vi "DSF.Shared.Configuration.Transfer.Get Engine Offset.vi"(11 "Transfer Configuration in":refnum<class "DSF.Shared.Configuration.Transfer.lvclass">) -> (2 "engine offset":u64, 3 "Transfer Configuration out":refnum<class "DSF.Shared.Configuration.Transfer.lvclass">)   [LabVIEW 2017, in "DSF.Engine.lvlib" / "DSF.Shared.Configuration.Transfer.lvclass"]
uses:
  DSF.Shared.Configuration.Transfer.lvclass
  DSF.Shared.Configuration.Transfer.lvclass/DSF.Shared.Configuration.Transfer.ctl
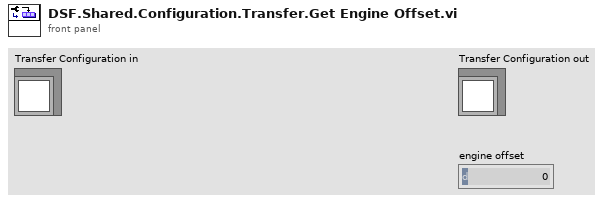
[diagram p1: front panel]
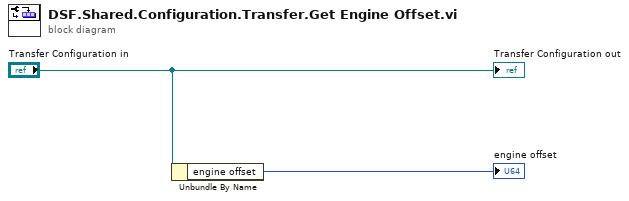
[diagram p0: block diagram]
diagram:
  n1 = Unbundle By Name("Transfer Configuration in") -> ("engine offset"=→"engine offset":u64)
  "Transfer Configuration out" <- "Transfer Configuration in"
